vi "getSerializedData.vi"(0 "reference":refnum<class "NoteNode.lvclass">, 5 "error in (no error)":errorcluster) -> (14 "reference out":refnum<class "NoteNode.lvclass">, 15 "parent":refnum<class "AbstractNode.lvclass">, 16 "children":refnum<class "AbstractNode.lvclass">[](array[class]), 17 "xmlOut":string, 19 "error out":errorcluster)   [LabVIEW 2012, in "NoteNode.lvclass"]
doc: "getSerializedData"
uses:
  <resource>/Framework/Providers/Open_GDS/UML/NoteNode_class/NoteNode.lvclass
  <resource>/Framework/Providers/Open_GDS/UML/AbstractNode_class/AbstractNode.lvclass
  <resource>/Framework/Providers/Open_GDS/UML/AbstractNode_class/ObjectReference.ctl
  <resource>/Framework/Providers/Open_GDS/UML/General/Rectangle/Rectangle Rectangle2D.ctl
  <resource>/Framework/Providers/Open_GDS/UML/MultiLineString_class/ObjectReference.ctl
  <resource>/Framework/Providers/Open_GDS/UML/MultiLineString_class/JustificationType.ctl
  <resource>/Framework/Providers/Open_GDS/UML/MultiLineString_class/MultiLineString.lvclass
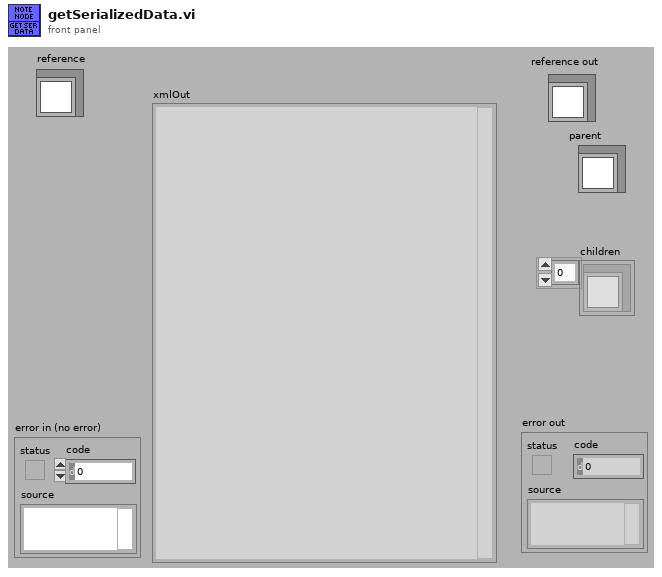
[diagram p1: front panel]
types:
  T1 = typedef "AbstractNode.lvclass/ObjectReference.ctl" = refnum<k1>
  T2 = typedef "Rectangle Rectangle2D.ctl" = cluster{"x":dbl, "y":dbl, "width":dbl, "height":dbl}
  T3 = typedef "MultiLineString.lvclass/ObjectReference.ctl" = refnum<k1>
  T4 = cluster{"Base class":cluster{"Base class":cluster{"parent":T1, "children":T1[], "Hidden":bool}, "bounds":T2}, "DEFAULT_WIDTH":i32, "DEFAULT_HEIGHT":i32, "DEFAULT_COLOR":u32, "FOLD_X":i32, "FOLD_Y":i32, "color":u32, "text":T3, "pointNodes":T1[]}
  T5 = typedef "MultiLineString.lvclass/JustificationType.ctl" = enum16{"LEFT", "CENTER", "RIGHT"}
  T6 = typedef "NoteNode.lvclass/ObjectAttributes.ctl" = cluster{"Base class":T7, "DEFAULT_WIDTH":i32, "DEFAULT_HEIGHT":i32, "DEFAULT_COLOR":u32, "FOLD_X":i32, "FOLD_Y":i32, "color":u32, "text":refnum<class "MultiLineString.lvclass">, "pointNodes":refnum<class "AbstractNode.lvclass">[]}
  T7 = typedef "RectangularNode.lvclass/ObjectAttributes.ctl" = cluster{"Base class":T8, "bounds":T2}
  T8 = typedef "AbstractNode.lvclass/ObjectAttributes.ctl" = cluster{"parent":refnum<class "AbstractNode.lvclass">, "children":refnum<class "AbstractNode.lvclass">[], "Hidden":bool}
  T9 = cluster{"Attributes":cluster{"Base class":cluster{"Base class":cluster{"parent":T1, "children":T1[], "Hidden":bool}, "bounds":T2}, "DEFAULT_WIDTH":i32, "DEFAULT_HEIGHT":i32, "DEFAULT_COLOR":u32, "FOLD_X":i32, "FOLD_Y":i32, "color":u32, "text":T3, "pointNodes":T1[]}, string}
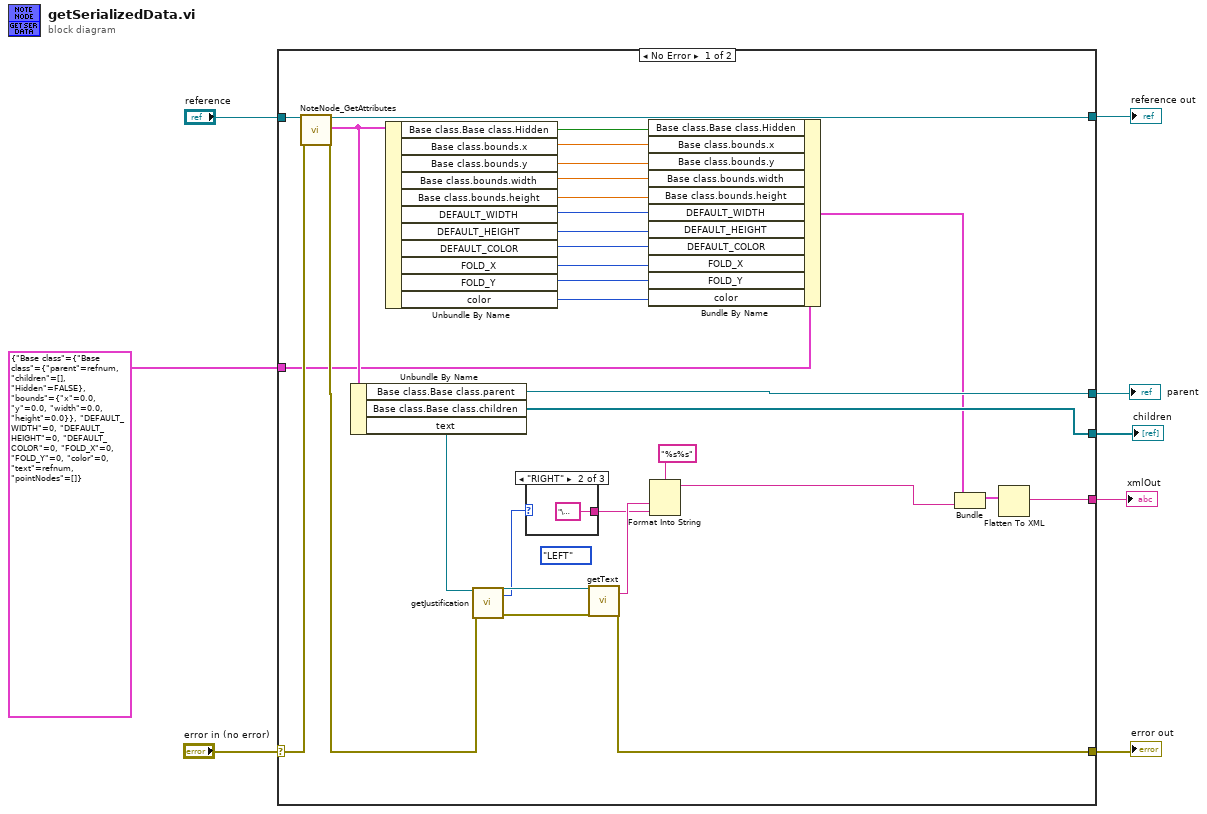
[diagram p0: block diagram]
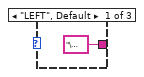
[diagram p2: hidden frame]
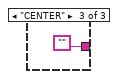
[diagram p3: hidden frame]
diagram:
  n1 = case shown="No Error" "error in (no error)" {
    selector: "error in (no error)" -> [w39 w43]
    tunnel: "reference" -> [w38 w44]
    tunnel: [w35 w43] -> w6
    tunnel: [w37 w44] -> w5
    tunnel: [w34 _] -> w4
    tunnel: [w33 _] -> w3
    tunnel: [w32 _] -> w2
    tunnel: T4 {"Base class"={"Base class"={"parent"=refnum, "children"=[], "Hidden"=FALSE}, "bounds"={"x"=0.0, "y"=0.0, "width"=0.0, "height"=0.0}}, "DEFAULT_WIDTH"=0, "DEFAULT_HEIGHT"=0, "DEFAULT_COLOR"=0, "FOLD_X"=0, "FOLD_Y"=0, "color"=0, "text"=refnum, "pointNodes"=[]} ("Attributes") -> [w21 _]
    frame No Error {
      (unwired) JustificationType."LEFT" ("justification")
      n2 = call <resource>:"NoteNode_GetAttributes.vi"("reference in"=w38, "error in (no error)"=w39) -> ("reference out"=w37:refnum<class "NoteNode.lvclass">, "Attributes"=w22:T6, "error out"=w29:errorcluster)  [unwired: 15 out]
      n3 = Unbundle By Name(w22) -> ("Base class.Base class.parent"=w34:refnum<class "AbstractNode.lvclass">, "Base class.Base class.children"=w33:refnum<class "AbstractNode.lvclass">[], "text"=w28:refnum<class "MultiLineString.lvclass">)
      n4 = Unbundle By Name(w22) -> ("Base class.Base class.Hidden"=w9:bool, "Base class.bounds.x"=w20:dbl, "Base class.bounds.y"=w19:dbl, "Base class.bounds.width"=w18:dbl, "Base class.bounds.height"=w17:dbl, "DEFAULT_WIDTH"=w16:i32, "DEFAULT_HEIGHT"=w15:i32, "DEFAULT_COLOR"=w14:u32, "FOLD_X"=w13:i32, "FOLD_Y"=w12:i32, "color"=w11:u32)
      n5 = call <resource>:"getJustification.vi"("reference"=w28, "error in (no error)"=w29) -> ("reference out"=w31:refnum<class "MultiLineString.lvclass">, "justification"=w24:T5, "error out"=w30:errorcluster)  [unwired: 15 out]
      n6 = case shown="\"RIGHT\"" w24 {
        tunnel: ["\u0001" "\u0003" ""] -> w23
        frame "LEFT", Default {
        }
        frame "RIGHT" {
        }
        frame "CENTER" {
        }
      }
      n7 = call-dynamic "getText.vi"("reference"=w31, "error in (no error)"=w30) -> ("text"=w26:string, "error out"=w35:errorcluster)  [unwired: 16 out]
      n8 = Bundle By Name(cluster=w21, "Base class.Base class.Hidden"=w9, "Base class.bounds.x"=w20, "Base class.bounds.y"=w19, "Base class.bounds.width"=w18, "Base class.bounds.height"=w17, "DEFAULT_WIDTH"=w16, "DEFAULT_HEIGHT"=w15, "DEFAULT_COLOR"=w14, "FOLD_X"=w13, "FOLD_Y"=w12, "color"=w11) -> (w10:T4)
      n9 = Format Into String(format string="%s%s", w26, w23) -> (resulting string=w25:string)  [unwired: 2 in, 1 out]
      n10 = Bundle("Attributes"=w10, w25) -> (w36:T9)  [unwired: 1 out]
      n11 = Flatten To XML(anything=w36) -> (xml string=w32:string)
    }
    frame Error {
    }
  }
  "reference out" <- w5
  "error out" <- w6
  "parent" <- w4
  "children" <- w3
  "xmlOut" <- w2
